vi "setCommandValveAngle02.vi"(1 "error in (no error)":errorcluster, 2 "angle(deg)":dbl) -> (0 "error out":errorcluster)   [LabVIEW 2011]
panel:
  out "concatenated string":string
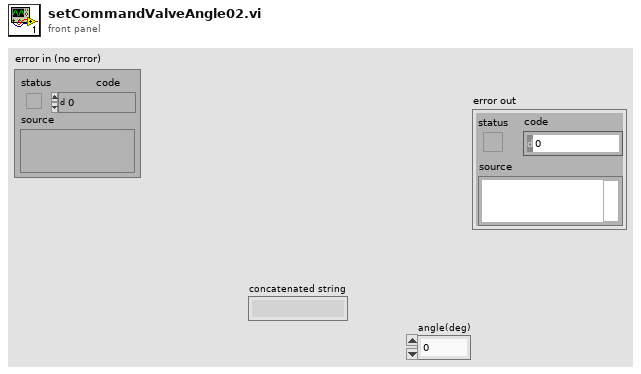
[diagram p1: front panel]
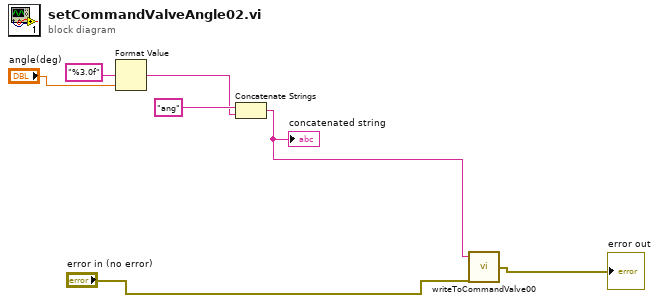
[diagram p0: block diagram]
diagram:
  n1 = Format Value(format string="%3.0f", value (0)="angle(deg)") -> (output string=w4:string)  [unwired: 1 in]
  n2 = Concatenate Strings("ang" ("string to write"), w4) -> (w2:string)
  "concatenated string" <- w2
  n3 = call "writeToCommandValve00.vi"("error in (no error)"="error in (no error)", "String"=w2) -> ("error out"=→"error out":errorcluster)  [unwired: 1 in]
